vi "TriVert-in-Box test.vi"(1 "Triangle":T1, 2 "Box":T2) -> (0 "Vertex is inside box":bool)   [LabVIEW 2014]
uses:
  Typedefs/TreeNodeBox.ctl
  Typedefs/Quad.ctl
  Typedefs/Triangle.ctl
panel:
  # "PN 17/01/2015"
  # "Vertices"
  # "Edges"
  # "Unit normal"
  # "pre-store"
  # "Vertices"
  # "Edges"
  # "Unit normal"
  # "Edge unit normals"
  # "Vertices"
  # "Edges"
  # "Unit normal"
  # "Edge unit normals"
  # "Vertices"
  # "Edges"
  # "Unit normal"
  # "Edge unit normals"
  # "Vertices"
  # "Edges"
  # "Unit normal"
  # "Edge unit normals"
  # "Vertices"
  # "Edges"
  # "Unit normal"
  # "Edge unit normals"
  # "Vertices"
  # "Edges"
  # "Unit normal"
  # "Edge unit normals"
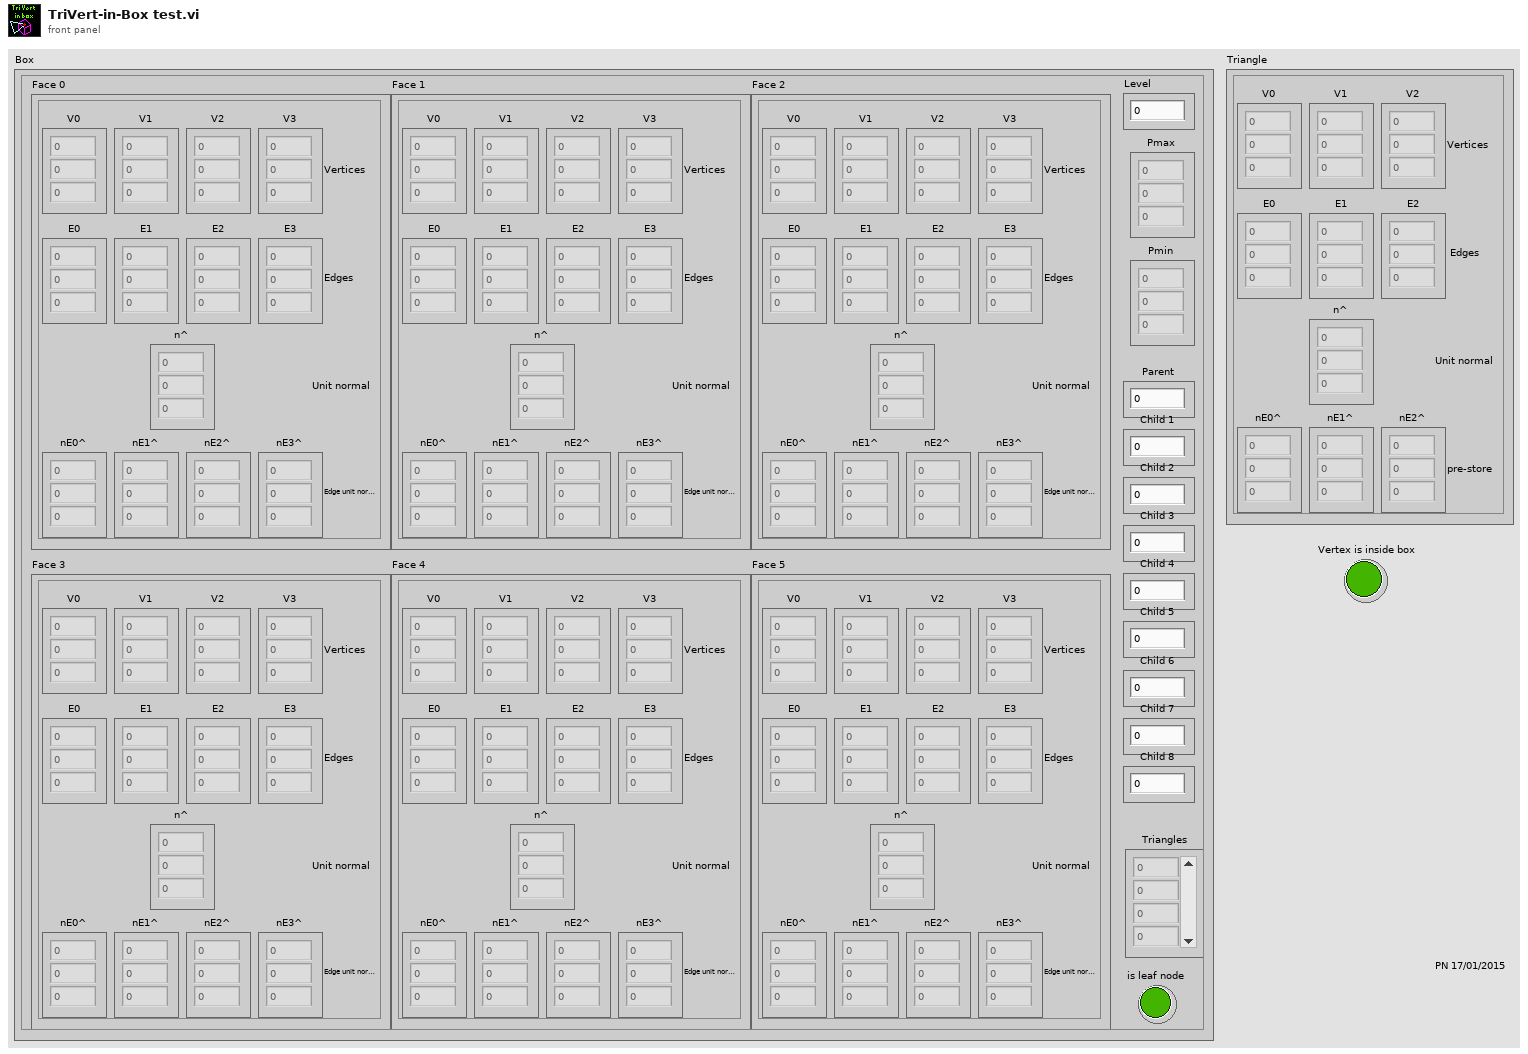
[diagram p1: front panel]
types:
  T1 = typedef "Triangle.ctl" = cluster{"V0":sgl[], "V1":sgl[], "V2":sgl[], "E0":sgl[], "E1":sgl[], "E2":sgl[], "n^":sgl[], "nE0^":sgl[], "nE1^":sgl[], "nE2^":sgl[]}
  T2 = typedef "TreeNodeBox.ctl" = cluster{"Face 0":T3, "Face 1":T3, "Face 2":T3, "Face 3":T3, "Face 4":T3, "Face 5":T3, "Level":i32, "Pmax":sgl[], "Pmin":sgl[], "Parent":i32, "Child 1":i32, "Child 2":i32, "Child 3":i32, "Child 4":i32, "Child 5":i32, "Child 6":i32, "Child 7":i32, "Child 8":i32, "Triangles":i32[], "is leaf node":bool}
  T3 = typedef "Quad.ctl" = cluster{"V0":sgl[], "V1":sgl[], "V2":sgl[], "V3":sgl[], "E0":sgl[], "E1":sgl[], "E2":sgl[], "E3":sgl[], "n^":sgl[], "nE0^":sgl[], "nE1^":sgl[], "nE2^":sgl[], "nE3^":sgl[]}
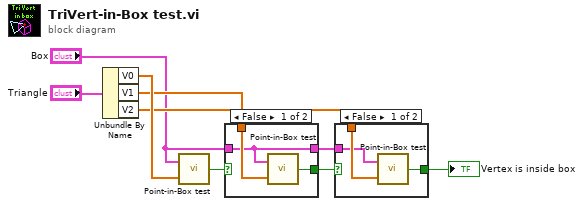
[diagram p0: block diagram]
diagram:
  n1 = Unbundle By Name("Triangle") -> ("V0"=w8:sgl[], "V1"=w6:sgl[], "V2"=w3:sgl[])
  n2 = call "Point-in-Box test.vi"("Point"=w8, "Box"="Box") -> ("Point is inside box"=w7:bool)
  n3 = case shown="False" w7 {
    selector: w7 -> [_ w14]
    tunnel: [w11 w14] -> w5
    tunnel: w6 -> [w12 _]
    tunnel: "Box" -> [w10 w13]
    tunnel: [w10 w13] -> w1
    frame False {
      n4 = call "Point-in-Box test.vi"("Point"=w12, "Box"=w10) -> ("Point is inside box"=w11:bool)
    }
    frame True {
    }
  }
  n5 = case shown="False" w5 {
    selector: w5 -> [_ w18]
    tunnel: [w16 w18] -> w4
    tunnel: w3 -> [w17 _]
    tunnel: w1 -> [w15 _]
    frame False {
      n6 = call "Point-in-Box test.vi"("Point"=w17, "Box"=w15) -> ("Point is inside box"=w16:bool)
    }
    frame True {
    }
  }
  "Vertex is inside box" <- w4
